vi "test-DiffDriveSim-convergence.vi"() -> (3 "Test Passed":bool)   [LabVIEW 2019]
uses:
  <vilib>/Rock Robotics/WPI/ThirdParty/JAS_Junk/TrajLib/DCMOTOR.CTL
  <vilib>/Rock Robotics/WPI/ThirdParty/JAS_Junk/TrajLib/LINEAR_SYSTEM.ctl
  <vilib>/Analysis/Matrix/Datatypes/RealMatrix.ctl
  <vilib>/Rock Robotics/WPI/ThirdParty/JAS_Junk/TrajLib/DIFF_DRIVE_TRAIN_SIM.ctl
  <vilib>/Rock Robotics/WPI/ThirdParty/JAS_Junk/TrajLib/POSE2D.ctl
  <vilib>/Rock Robotics/WPI/ThirdParty/JAS_Junk/TrajLib/TRANSLATION2D.ctl
  <vilib>/Rock Robotics/WPI/ThirdParty/JAS_Junk/TrajLib/ROTATION2D.ctl
  <vilib>/Rock Robotics/WPI/ThirdParty/JAS_Junk/TrajLib/DIFF_DRIVE_ToughBoxMini_MotorChoice_ENUM.ctl
  <vilib>/Rock Robotics/WPI/ThirdParty/JAS_Junk/TrajLib/TRAJECTORY_SPLINE_TYPE_ENUM.ctl
  <vilib>/Rock Robotics/WPI/ThirdParty/JAS_Junk/TrajLib/Translation2d_Create.vi
  <vilib>/Rock Robotics/WPI/ThirdParty/JAS_Junk/TrajLib/Rotation2d_CreateAngle.vi
  <vilib>/Rock Robotics/WPI/ThirdParty/JAS_Junk/TrajLib/MatBuilder_Create.vi
  <vilib>/Rock Robotics/SystemInterfaces/NetworkCommunication/NetComm_UsageReport_report.vi
  <vilib>/Rock Robotics/WPI/ThirdParty/JAS_Junk/TrajLib/DiffDriveKinematicsConstraint_New.vi
  <vilib>/Rock Robotics/WPI/ThirdParty/JAS_Junk/TrajLib/LinearSystem_New.vi
  <vilib>/Rock Robotics/WPI/ThirdParty/JAS_Junk/TrajLib/MatBuilder_Fill.vi
  <vilib>/Rock Robotics/WPI/ThirdParty/JAS_Junk/TrajLib/MatrixHelper_Zero.vi
  <vilib>/Rock Robotics/WPI/ThirdParty/JAS_Junk/TrajLib/Ramsete_New_B_Z.vi
  <vilib>/Rock Robotics/WPI/ThirdParty/JAS_Junk/TrajLib/Ramsete_SetTolerance.vi
  <vilib>/Rock Robotics/WPI/ThirdParty/JAS_Junk/TrajLib/Pose2d_New.vi
  <vilib>/Rock Robotics/WPI/ThirdParty/JAS_Junk/TrajLib/Conv_AngleRadians_Heading.vi
  <vilib>/Rock Robotics/WPI/ThirdParty/JAS_Junk/TrajLib/Ramsete_SetEnabled.vi
  <vilib>/Rock Robotics/WPI/ThirdParty/JAS_Junk/TrajLib/MatrixHelper_CoerceSize.vi
  <vilib>/Rock Robotics/WPI/ThirdParty/JAS_Junk/TrajLib/Util_LibraryGlobals.vi
  <vilib>/Rock Robotics/WPI/ThirdParty/JAS_Junk/TrajLib/DiffDriveTrainSim_GetDynamics.vi
  <vilib>/Rock Robotics/WPI/ThirdParty/JAS_Junk/TrajLib/Ramsete_Diff_DO_SI.vi
  <vilib>/Rock Robotics/WPI/ThirdParty/JAS_Junk/TrajLib/DiffWheel_Normalize.vi
  <vilib>/Rock Robotics/WPI/ThirdParty/JAS_Junk/TrajLib/Trajectory_Library.lvlib
  <vilib>/Analysis/Matrix/NI_Matrix.lvlib
panel:
  in  "Tab Control":T1(tab)
  out "SP Chart":T2(graph)
  out "XY Graph":cluster{dbl[], dbl[]}[](graph)
  out "Left Motor Vel (PV)":dbl format="%20.3f"
  out "Right Motor Vel (PV)":dbl format="%20.3f"
  out "Motor Amps":cluster{"Voltage":dbl}(graph)
  out "PV Chart":T2(graph)
  out "Motor Amps":dbl format="%20.3f"
  out "Sim Upd Err":bool
  out "Lin Sys Size Cooerced":bool
  out "AtReference":bool
  out "InvFF Error":bool
  out "SIM Pose":T3={"TRANSLATION"={"X"=0.0, "Y"=0.0}, "ROTATION"={"VALUE"=0.0, "COS"=1.0, "SIN"=0.0}} {"ROTATION"."SIN" format="%13.4f"; "ROTATION"."COS" format="%13.4f"; "ROTATION"."VALUE" format="%13.4f"; "TRANSLATION"."Y" format="%14.3f"; "TRANSLATION"."X" format="%14.3f"}
  out "m_Y":T6
  out "m_X":T6
  out "Ground Truth":T6
  out "RK4 Error":bool
  out "DiffDriveMotor":T7 {"Jr_KgM2" format="%13.5p"; "L_H" format="%13.5p"; "Kt_NMPerAmp" format="%13.5p"; "KvINV_RadPerSecPerVolt" format="%13.5p"; "R_Ohms" format="%13.5p"; "FreeSpeed_RadPerSec" format="%13.5p"; "FreeCurrent_Amps" format="%13.5p"; "StallCurrent_Amps" format="%13.5p"; "StallTorque_NM" format="%13.5p"; "nominalVoltage_Volts" format="%13.5p"}
  out "m_DiffDriveVel":T8
  out "Differential Drive Train Sim":T9 {"m_Motor"."Jr_KgM2" format="%13.5p"; "m_Motor"."L_H" format="%13.5p"; "m_Motor"."Kt_NMPerAmp" format="%13.5p"; "m_Motor"."KvINV_RadPerSecPerVolt" format="%13.5p"; "m_Motor"."R_Ohms" format="%13.5p"; "m_Motor"."FreeSpeed_RadPerSec" format="%13.5p"; "m_Motor"."FreeCurrent_Amps" format="%13.5p"; "m_Motor"."StallCurrent_Amps" format="%13.5p"; "m_Motor"."StallTorque_NM" format="%13.5p"; "m_Motor"."nominalVoltage_Volts" format="%13.5p"}
  # "<States,States>"
  # "<States,Inputs>"
  # "<Outputs,States>"
  # "<Outputs,Inputs>"
  # "<States, 1>"
  # "<Outputs, 1>"
  # "<Inputs, 1>"
  # "<Outputs, 1>"
  # "<States,States>"
  # "<States,Inputs>"
  # "<Outputs,States>"
  # "<Outputs,Inputs>"
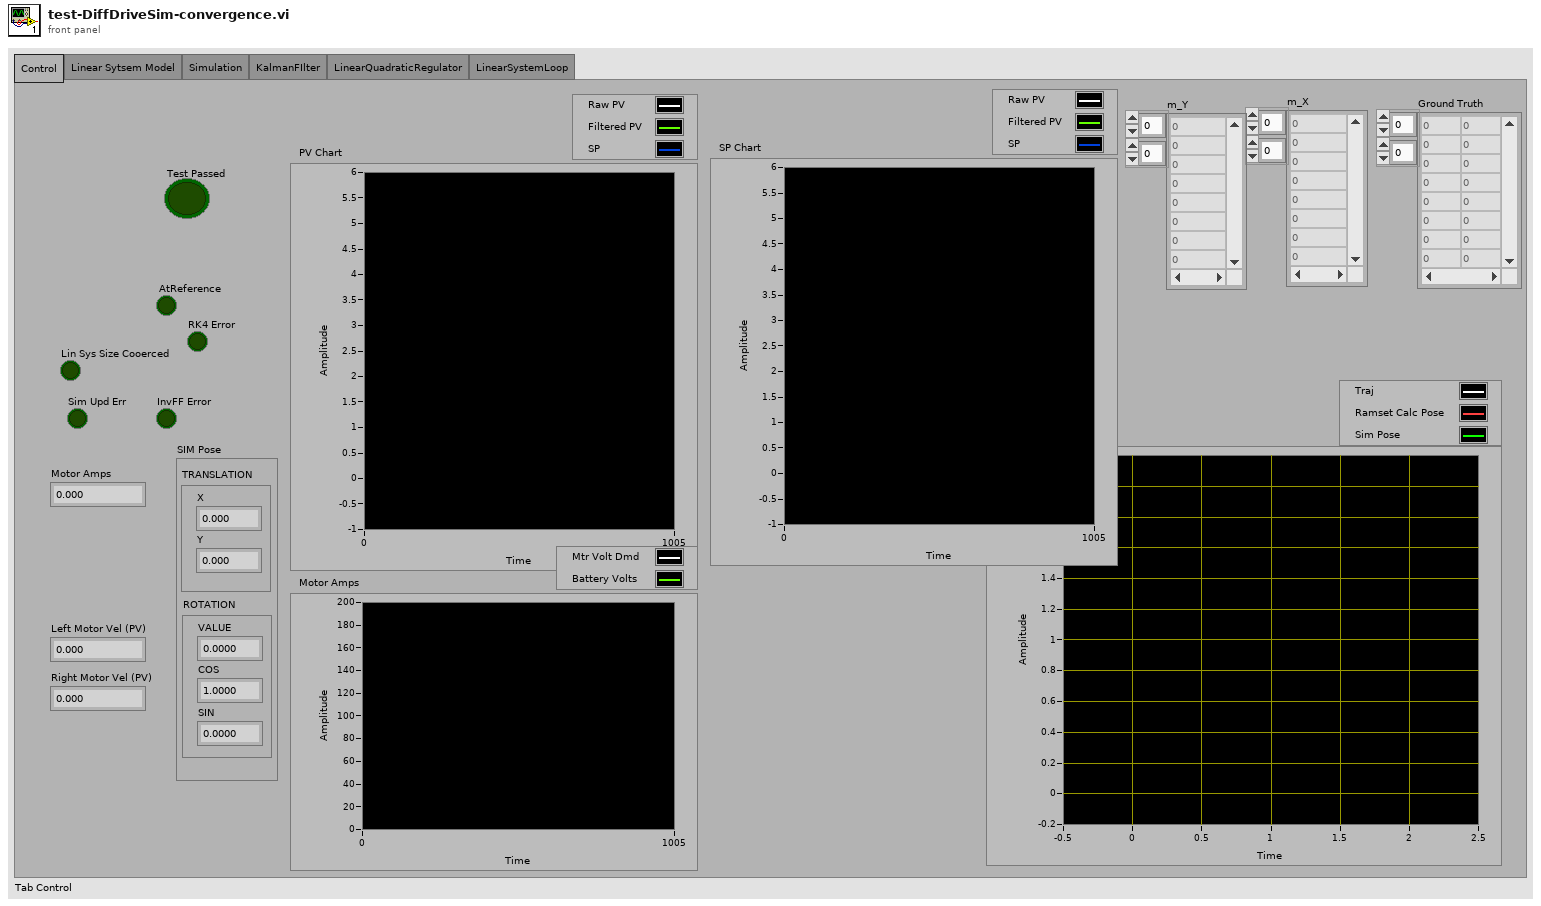
[diagram p1: front panel]
types:
  T1 = enum32{"Control", "Linear Sytsem Model", "Simulation", "KalmanFIlter", "LinearQuadraticRegulator", "LinearSystemLoop"}
  T2 = cluster{"LeftVelocity_M_Per_Sec":dbl, "RightVel_M_Per_Sec":dbl}
  T3 = typedef "Trajectory_Library.lvlib/POSE2D.ctl" = cluster{"TRANSLATION":T4, "ROTATION":T5}
  T4 = typedef "Trajectory_Library.lvlib/TRANSLATION2D.ctl" = cluster{"X":dbl, "Y":dbl}
  T5 = typedef "Trajectory_Library.lvlib/ROTATION2D.ctl" = cluster{"VALUE":dbl, "COS":dbl, "SIN":dbl}
  T6 = typedef "NI_Matrix.lvlib/RealMatrix.ctl" = dbl[][]
  T7 = typedef "Trajectory_Library.lvlib/DCMOTOR.CTL" = cluster{"nominalVoltage_Volts":dbl, "StallTorque_NM":dbl, "StallCurrent_Amps":dbl, "FreeCurrent_Amps":dbl, "FreeSpeed_RadPerSec":dbl, "R_Ohms":dbl, "KvINV_RadPerSecPerVolt":dbl, "Kt_NMPerAmp":dbl, "L_H":dbl, "Jr_KgM2":dbl}
  T8 = typedef "Trajectory_Library.lvlib/LINEAR_SYSTEM.ctl" = cluster{"m_A":T6, "m_B":T6, "m_C":T6, "m_D":T6, "States":i32, "Inputs":i32, "Outputs":i32}
  T9 = typedef "Trajectory_Library.lvlib/DIFF_DRIVE_TRAIN_SIM.ctl" = cluster{"m_Plant":T8, "m_X":T6, "m_Y":T6, "m_U":T6, "MeasureStdDev":T6, "m_Motor":T7, "m_OriginalGearing":dbl, "m_CurrentGearing":dbl, "m_WheelRadius_M":dbl, "m_RB":dbl}
  T10 = typedef "Trajectory_Library.lvlib/TRAJECTORY_SPLINE_TYPE_ENUM.ctl" = enum16{"Cubic", "Cubic With Weights", "Quintic", "Quintic With Weights"}
  T11 = typedef "Trajectory_Library.lvlib/DIFF_DRIVE_ToughBoxMini_MotorChoice_ENUM.ctl" = enum16{"One CIM Per Side", "Two CIM Per Side", "One MiniCIM Per Side", "Two Mini CIM Per Side", "Two Falcon Per Side", "Two NEO Per Side"}
  T12 = typedef "Trajectory_Library.lvlib/TRAJ_CONFIG.ctl" = cluster{"MaxVelocity":dbl, "Max Acceleration":dbl, "StartVelocity":dbl, "End Velocity":dbl, "Reversed":bool, "DiffDrKineConstntDefined":bool, "CentAcellConstntDefined":bool, "DiffDrVoltConstntDefined":bool, "DIFF_DRIVE_KINE_CONSTRAINT":T13, "CENTRIPETAL_ACCEL_CONSTRAINT":T15, "SwerveDrKineConstntDefined":bool, "SWERVE_DRIVE_KINE_CONSTRAINT":T16, "DIFF_DRIVE_VOLTAGE_CONSTRAINT":T18, "MECANUM_DRIVE_KINE_CONSTRAINT":T20, "MecanumDrKineConstntDefined":bool}
  T13 = typedef "Trajectory_Library.lvlib/TRAJ_CONSTRAINT_DIIF_DRIVE_KINEMATICS.ctl" = cluster{"Max Speed (M/S)":dbl, "DIFF_DRIVE_KINEMATICS":T14, "Max Accel (M/S2)":dbl}
  T14 = typedef "Trajectory_Library.lvlib/DIFF_DRIVE_KINEMATICS.ctl" = cluster{"TrackWidth_Meters":dbl}
  T15 = typedef "Trajectory_Library.lvlib/TRAJ_CONSTRAINT_CENTRIPETAL_ACCEL.ctl" = cluster{"Max Cent Accel":dbl}
  T16 = typedef "Trajectory_Library.lvlib/TRAJ_CONSTRAINT_SWERVE_DRIVE_KINEMATICS.ctl" = cluster{"Max Speed (M/S)":dbl, "SwerveKinematics":T17}
  T17 = typedef "Trajectory_Library.lvlib/SWERVE_DRIVE_KINEMATICS.ctl" = cluster{"NumModules":i32, "InverseKinematics":T6, "ForwardKinematics":T6, "Modules":T4[], "PrevCoR":T4}
  T18 = typedef "Trajectory_Library.lvlib/TRAJ_CONSTRAINT_DIIF_DRIVE_VOLTAGE.ctl" = cluster{"Max Voltage":dbl, "DIFF_DRIVE_KINEMATICS":T14, "SIMPLE_MOTOR_FF":T19}
  T19 = typedef "Trajectory_Library.lvlib/SIMPLE_MOTOR_FF.ctl" = cluster{"Ks":dbl, "Kv":dbl, "Ka":dbl}
  T20 = typedef "Trajectory_Library.lvlib/TRAJ_CONSTRAINT_MECA_DRIVE_KINEMATICS.ctl" = cluster{"Max Speed (M/S)":dbl, "MECA_DRIVE_KINEMATICS":T21}
  T21 = typedef "Trajectory_Library.lvlib/MECA_DRIVE_KINEMATICS.ctl" = cluster{"FrontLeft":T4, "FrontRight":T4, "RearLeft":T4, "RearRight":T4, "InverseKinematics":T6, "ForwardKinematics":T6, "PrevCoR":T4}
  T22 = typedef "Trajectory_Library.lvlib/WEIGHTED_WAYPOINT.ctl" = cluster{"TRANSLATION":T4, "ROTATION":T5, "SCALAR":dbl}
  T23 = typedef "Trajectory_Library.lvlib/TRAJECTORY.ctl" = cluster{"TotalTImeSecs":dbl, "States":T24[]}
  T24 = typedef "Trajectory_Library.lvlib/TRAJ_STATE.ctl" = cluster{"TimeSeconds":dbl, "Velocity":dbl, "Acceleration":dbl, "POSE":T3, "Curvature":dbl}
  T25 = typedef "Trajectory_Library.lvlib/LINEAR_PLANT_INV_FF.ctl" = cluster{"m_R":T6, "m_Uff":T6, "m_B":T6, "m_A":T6, "States":i32, "Inputs":i32}
  T26 = typedef "Trajectory_Library.lvlib/RAMSETE_EXE_TUNING.ctl" = cluster{"B":dbl, "Zeta":dbl, "X Tolerance M":dbl, "Y Tolerance M":dbl, "Heading Tolerance RAD":dbl, "Track Width M":dbl, "Max Speed M/S":dbl}
  T27 = cluster{"Left Speed Dmd M/S":dbl, "Right Speed Dmd M/S":dbl}
  T28 = cluster{"m_A":T6, "m_B":T6, "m_CurrentGearing":dbl, "m_OriginalGearing":dbl, "m_RB":dbl}
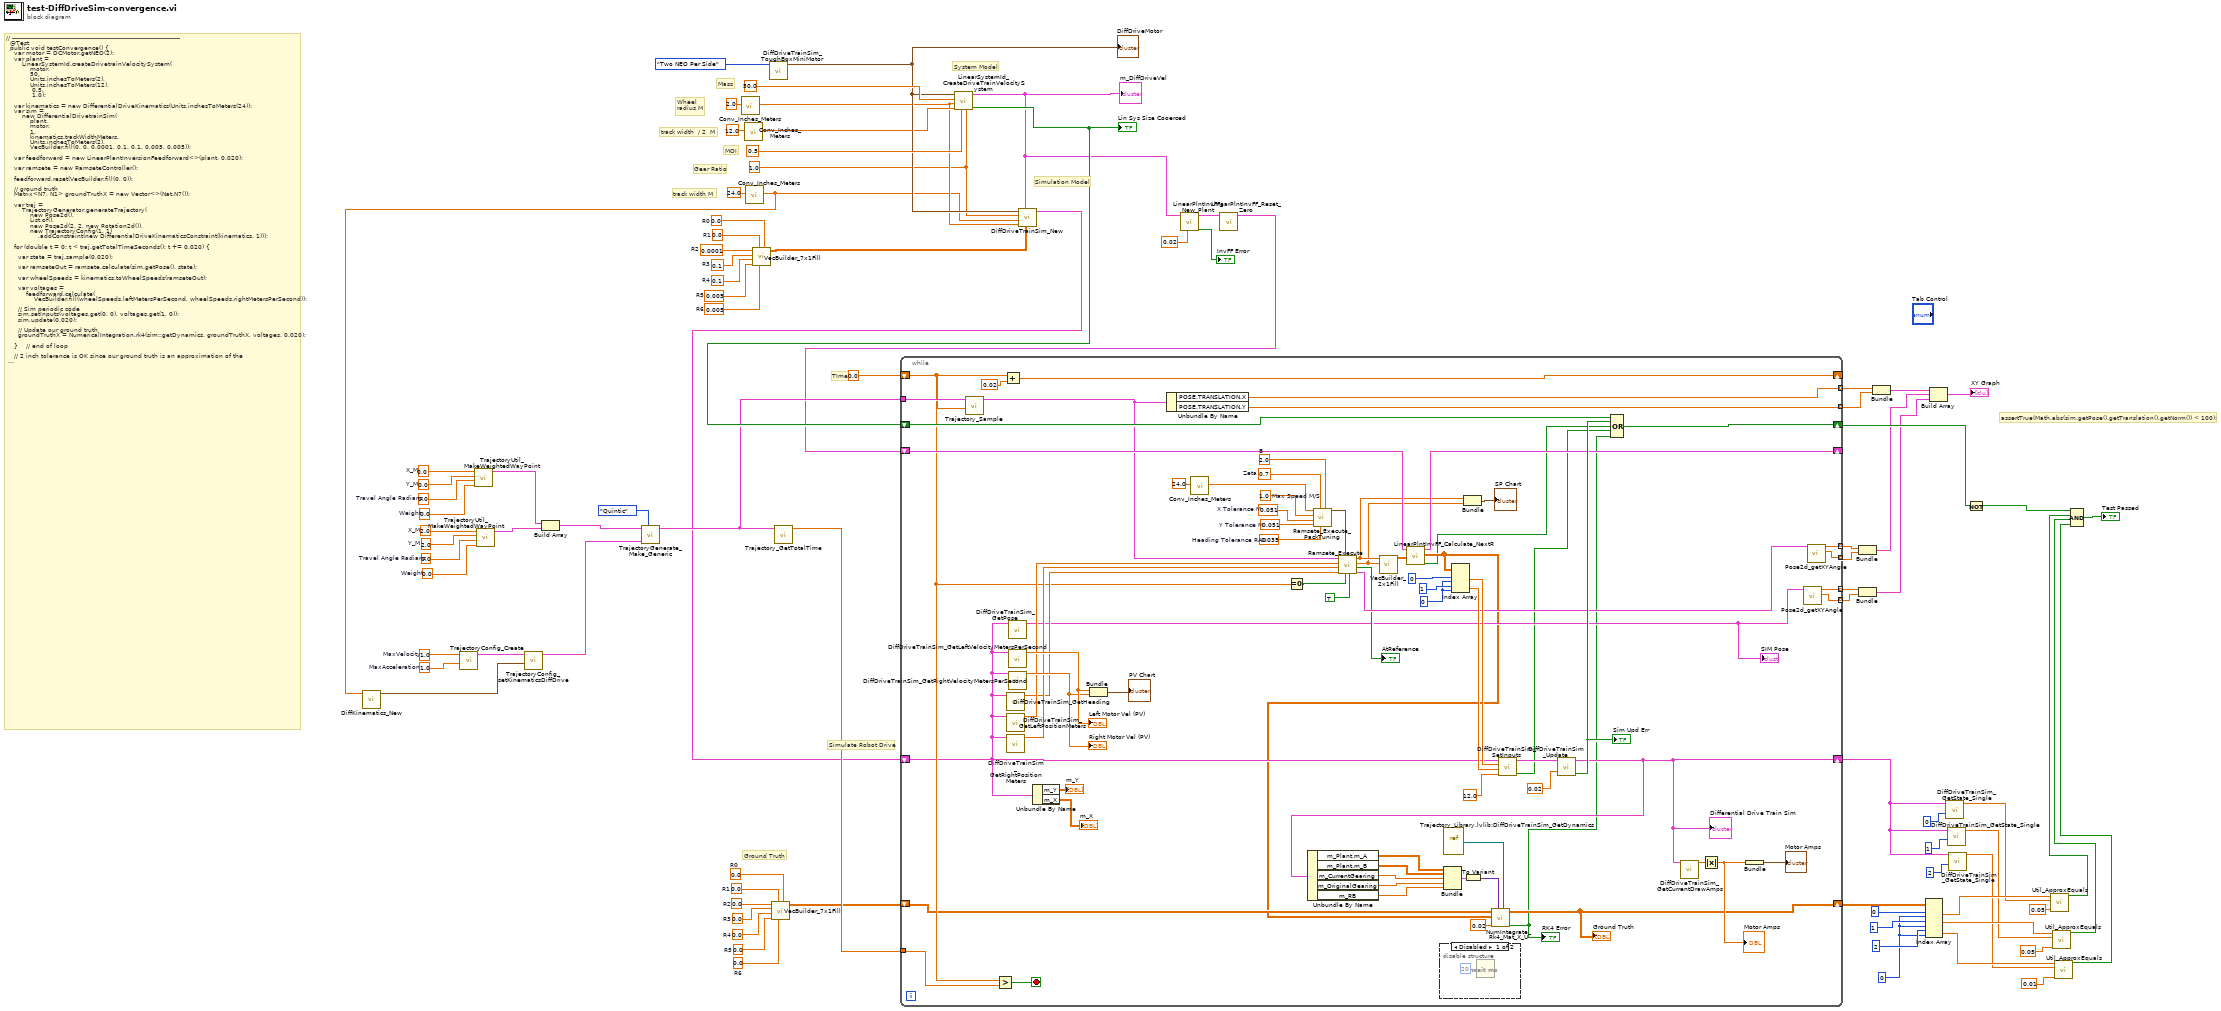
[diagram p0: block diagram]
diagram:
  w17 = 0 ("index (col)")
  w58 = 2.0  # X_M
  w57 = 2.0  # Y_M
  w56 = 0.0  # Travel Angle Radians
  w55 = 0.0  # Weight
  w54 = 0.0  # X_M
  w53 = 0.0  # Y_M
  w52 = 0.0  # Travel Angle Radians
  w51 = 0.0  # Weight
  w50 = 1.0  # MaxVelocity
  w49 = 1.0  # MaxAcceleration
  w66 = 0.0  # R6
  w65 = 0.0  # R5
  w64 = 0.0  # R4
  w63 = 0.0  # R3
  w62 = 0.0  # R2
  w61 = 0.0  # R1
  w60 = 0.0  # R0
  w78 = 0.005  # R6
  w77 = 0.005  # R5
  w76 = 0.1  # R4
  w75 = 0.1  # R3
  w74 = 0.0001  # R2
  w73 = 0.0  # R1
  w72 = 0.0  # R0
  w80 = 1.0 ("G")
  # "TIme"
  # "Ground Truth"
  # "// ------------------------------------------------------------------------------------\n  @Test\n  public void testConvergence() {\n    var motor = DCMotor.getNEO(2);\n    var plant =\n        LinearSystemId.createDrivetrainVelocitySystem(\n            motor, \n            50, \n            Units.inchesToMeters(2), \n            Units.inchesToMeters(12), \n             0.5, \n             1.0);\n\n    var kinematics = new DifferentialDriveKinematics(Units.inchesToMeters(24));\n    var sim =\n        new DifferentialDrivetrainSim(\n            plant,\n            motor,\n            1,\n            kinematics.trackWidthMeters,\n            Units.inchesToMeters(2),\n            VecBuilder.fill(0, 0, 0.0001, 0.1, 0.1, 0.005, 0.005));\n\n    var feedforward = new LinearPlantInversionFeedforward<>(plant, 0.020);\n\n    var ramsete = new RamseteController();\n\n    feedforward.reset(VecBuilder.fill(0, 0));\n\n    // ground truth\n    Matrix<N7, N1> groundTruthX = new Vector<>(Nat.N7());\n\n    var traj =\n        TrajectoryGenerator.generateTrajectory(\n            new Pose2d(),\n            List.of(),\n            new Pose2d(2, 2, new Rotation2d()),\n            new TrajectoryConfig(1, 1)\n                .addConstraint(new DifferentialDriveKinematicsConstraint(kinematics, 1)));\n\n    for (double t = 0; t < traj.getTotalTimeSeconds(); t += 0.020) {\n\n      var state = traj.sample(0.020);\n\n      var ramseteOut = ramsete.calculate(sim.getPose(), state);\n\n      var wheelSpeeds = kinematics.toWheelSpeeds(ramseteOut);\n\n      var voltages =\n          feedforward.calculate(\n              VecBuilder.fill(wheelSpeeds.leftMetersPerSecond, wheelSpeeds.rightMetersPerSecond));\n\n      // Sim periodic code\n      sim.setInputs(voltages.get(0, 0), voltages.get(1, 0));\n      sim.update(0.020);\n\n      // Update our ground truth\n      groundTruthX = NumericalIntegration.rk4(sim::getDynamics, groundTruthX, voltages, 0.020);\n\n    }    // end of loop\n\n    // 2 inch tolerance is OK since our ground truth is an approximation of the\n    // ODE solution using RK4 anyway\n    assertEquals(\n        groundTruthX.get(DifferentialDrivetrainSim.State.kX.value, 0),\n        sim.getState(DifferentialDrivetrainSim.State.kX),\n        0.05);\n    assertEquals(\n        groundTruthX.get(DifferentialDrivetrainSim.State.kY.value, 0),\n        sim.getState(DifferentialDrivetrainSim.State.kY),\n        0.05);\n    assertEquals(\n        groundTruthX.get(DifferentialDrivetrainSim.State.kHeading.value, 0),\n        sim.getState(DifferentialDrivetrainSim.State.kHeading),\n        0.01);\n  }\n\n\n}"
  # "assertTrue(Math.abs(sim.getPose().getTranslation().getNorm()) < 100);"
  # "track width M"
  # "Gear Ratio"
  # "Wheel\nradius M"
  # "track width  / 2  M"
  # "MOI"
  # "Simulation Model"
  # "System Model"
  # "Mass"
  # "Simulate Robot Drive"
  n1 = call <vilib>:"TrajectoryConfig_Create.vi"("MaxAcceleration"=w49, "MaxVelocity"=w50) -> ("TRAJECTORY_CONFIG"=w43:T12)  [unwired: 9 in]
  n2 = call <vilib>:"TrajectoryUtil_MakeWeightedWayPoint.vi"("Weight"=w51, "Travel Angle Radians"=w52, "Y_M"=w53, "X_M"=w54) -> ("WEIGHTED_WAYPOINT"=w46:T22)  [unwired: 7 in]
  n3 = call <vilib>:"TrajectoryUtil_MakeWeightedWayPoint.vi"("Weight"=w55, "Travel Angle Radians"=w56, "Y_M"=w57, "X_M"=w58) -> ("WEIGHTED_WAYPOINT"=w59:T22)  [unwired: 7 in]
  n4 = Build Array(w46, w59) -> (w47:T22[])
  n5 = call <vilib>:"Conv_Inches_Meters.vi"("INCH"=2.0) -> ("Meters"=w81:dbl)  [unwired: 10 in]
  n6 = call <vilib>:"Conv_Inches_Meters.vi"("INCH"=12.0) -> ("Meters"=w82:dbl)  [unwired: 10 in]
  n7 = call <vilib>:"Conv_Inches_Meters.vi"("INCH"=24.0) -> ("Meters"=w45:dbl)  [unwired: 10 in]
  n8 = call <vilib>:"DiffKinematics_New.vi"("TrackWidth_Meters"=w45) -> ("DIFF_DRIVE_KINEMATICS"=w44:T14)  [unwired: 10 in]
  n9 = call <vilib>:"TrajectoryConfig_setKinematicsDiffDrive.vi"("DIFF_DRIVE_KINEMATICS"=w44, "inTRAJECTORY_CONFIG"=w43) -> ("outTRAJECTORY_CONFIG"=w42:T12)  [unwired: 9 in]
  n10 = call <vilib>:"TrajectoryGenerate_Make_Generic.vi"("Spline Type"=TRAJECTORY_SPLINE_TYPE_ENUM."Quintic", "traj_config"=w42, "WeightedWayPoints"=w47) -> ("TRAJECTORY"=w36:T23)  [unwired: 7 in, 1 out]
  n11 = call <vilib>:"VecBuilder_7x1Fill.vi"("R0"=w72, "R6"=w78, "R1"=w73, "R5"=w77, "R4"=w76, "R3"=w75, "R2"=w74) -> ("output matrix"=w71:T6)  [unwired: 4 in]
  n12 = call <vilib>:"DiffDriveTrainSim_ToughBoxMiniMotor.vi"("ToughBoxMiniMotor"=DIFF_DRIVE_ToughBoxMini_MotorChoice_ENUM."Two NEO Per Side") -> ("DriveMotor"=w83:T7)  [unwired: 10 in]
  "DiffDriveMotor" <- w83
  n13 = call <vilib>:"VecBuilder_7x1Fill.vi"("R0"=w60, "R6"=w66, "R1"=w61, "R5"=w65, "R4"=w64, "R3"=w63, "R2"=w62) -> ("output matrix"=w22:T6)  [unwired: 4 in]
  n14 = call <vilib>:"Trajectory_GetTotalTime.vi"("TRAJECTORY"=w36) -> ("TotalTime_Sec"=w35:dbl)  [unwired: 10 in]
  n15 = call <vilib>:"LinearSystemId_CreateDriveTrainVelocitySystem.vi"("G"=w80, "JKgMetersSquared"=0.5 ("Mass_Kg"), "rbMeters"=w82, "rMeters"=w81, "MassKg"=50.0 ("Mass_Kg"), "Motor"=w83) -> ("Size Coerced"=w70:bool, "Linearsystem"=w40:T8)  [unwired: 4 in]
  "m_DiffDriveVel" <- w40
  "Lin Sys Size Cooerced" <- w70
  n16 = call <vilib>:"DiffDriveTrainSim_New.vi"("MeasurementStdDev"=w71, "DriveTrainPlant"=w40, "WheelRadius_M"=w81, "TrackWidth_M"=w45, "Gearing"=w80, "DriveMotor"=w83) -> ("DiffDriveTrainSim"=w33:T9)  [unwired: 5 in]
  n17 = call <vilib>:"LinearPlntInvFF_New_Plant.vi"("dT_Seconds"=0.02, "Plant"=w40) -> ("Error"=→"InvFF Error":bool, "Linear Plnt Inversion FF"=w38:T25)  [unwired: 8 in]
  n18 = call <vilib>:"LinearPlntInvFF_Reset_Zero.vi"("Input Linear Plant Inv FF"=w38) -> ("Output Linear Plant Inv FF"=w34:T25)  [unwired: 10 in]
  n19 = while {
    shift-right: [w104] -> w7
    shift-left: w33 -> [w107]
    shift-right: [w150] -> w69
    shift-left: w70 -> [w151]
    tunnel: w36 -> [w139]
    shift-right: [w147] -> _
    shift-left: 0.0 -> [w115]
    tunnel: w35 -> [w149]
    shift-right: [w133] -> _
    shift-left: w34 -> [w135]
    tunnel: [w124] -> w32 mode=indexing
    tunnel: [w123] -> w31 mode=indexing
    tunnel: [w122] -> w30 mode=indexing
    tunnel: [w121] -> w29 mode=indexing
    tunnel: [w109] -> w25 mode=indexing
    tunnel: [w108] -> w24 mode=indexing
    shift-right: [w92] -> w21
    shift-left: w22 -> [w95]
    stop <- w156 stop-if-true
    w128 = 0 ("index (col)")
    w146 = 1.0  # Max Speed M/S
    w145 = 0.051  # X Tolerance M
    w144 = 0.051  # Y Tolerance M
    w143 = 0.7  # Zeta
    w142 = 0.035  # Heading Tolerance RAD
    w141 = 2.0  # B
    n20 = call <vilib>:"Trajectory_Sample.vi"("Time"=w115, "InputTRAJECTORY"=w139) -> ("OutputTRAJ_STATE"=w125:T24)  [unwired: 9 in]
    n21 = Greater?(x=w115, y=w149) -> (0:w156:bool)
    n22 = Add(x=w115, y=0.02) -> (x+y=w147:dbl)
    n23 = call <vilib>:"DiffDriveTrainSim_GetHeading.vi"("DiffDriveTrainSim"=w107) -> ("Heading"=w136:dbl)  [unwired: 10 in]
    n24 = call <vilib>:"DiffDriveTrainSim_GetLeftPositionMeters.vi"("DiffDriveTrainSim"=w107) -> ("LeftPosition_Meters"=w138:dbl)  [unwired: 10 in]
    n25 = call <vilib>:"DiffDriveTrainSim_GetRightPositionMeters.vi"("DiffDriveTrainSim"=w107) -> ("RightPosition_Meters"=w137:dbl)  [unwired: 10 in]
    n26 = call <vilib>:"DiffDriveTrainSim_GetRightVelocityMetersPerSecond.vi"("DiffDriveTrainSim"=w107) -> ("RightVel_M_Per_Sec"=w154:dbl)  [unwired: 10 in]
    "Right Motor Vel (PV)" <- w154
    n27 = call <vilib>:"DiffDriveTrainSim_GetPose.vi"("DiffDriveTrainSim"=w107) -> ("Pose"=w110:T3)  [unwired: 10 in]
    "SIM Pose" <- w110
    n28 = call <vilib>:"DiffDriveTrainSim_GetLeftVelocityMetersPerSecond.vi"("DiffDriveTrainSim"=w107) -> ("LeftVelocity_M_Per_Sec"=w158:dbl)  [unwired: 10 in]
    "Left Motor Vel (PV)" <- w158
    n29 = Unbundle By Name(w107) -> ("m_Y"=→"m_Y":T6, "m_X"=→"m_X":T6)
    n30 = Bundle("LeftVelocity_M_Per_Sec"=w158, "RightVel_M_Per_Sec"=w154) -> (→"PV Chart":T2)  [unwired: 1 in]
    n31 = Unbundle By Name(w125) -> ("POSE.TRANSLATION.X"=w124:dbl, "POSE.TRANSLATION.Y"=w123:dbl)
    n32 = call <vilib>:"Conv_Inches_Meters.vi"("INCH"=24.0) -> ("Meters"=w113:dbl)  [unwired: 10 in]
    n33 = Equal To 0?(x=w115) -> (x = 0?=w116:bool)
    n34 = call <vilib>:"Ramsete_Execute_PackTuning.vi"("B"=w141, "Heading Tolerance RAD"=w142, "Zeta"=w143, "Y Tolerance M"=w144, "X Tolerance M"=w145, "Max Speed M/S"=w146, "Track Width M"=w113) -> ("RAMSETE_EXE_TUNING"=w140:T26)  [unwired: 4 in]
    n35 = call <vilib>:"Ramsete_Execute.vi"("Enabled"=TRUE, "Reset"=w116, "RAMSETE_EXE_TUNING"=w140, "Gyro-Radians\n(Inc counterclockwise)"=w136, "RightDist-Meters"=w137, "LeftDist-Meters"=w138, "TRAJ_STATE"=w125) -> ("CurrentRelativePose"=w112:T3, "AtReference"=→"AtReference":bool, "Right Speed Dmd M/S"=w118:dbl, "Left Speed Dmd M/S"=w119:dbl)  [unwired: 1 out]
    n36 = call <vilib>:"VecBuilder_2x1Fill.vi"("R1"=w118, "R0"=w119) -> ("output matrix"=w134:T6)  [unwired: 9 in]
    n37 = call <vilib>:"LinearPlntInvFF_Calculate_NextR.vi"("NextR"=w134, "Input Linear Plant Inv FF"=w135) -> ("Error"=w91:bool, "Uff"=w94:T6, "Output Linear Plant Inv FF"=w133:T25)  [unwired: 7 in]
    n38 = disable-structure shown="Disabled" {
      frame Disabled {
        n39 = Wait (ms)(milliseconds to wait=u32 20) -> ()  [unwired: 1 out]
      }
      frame Enabled {
      }
    }
    n40 = vi-ref "Trajectory_Library.lvlib:DiffDriveTrainSim_GetDynamics.vi"() -> (w96:refnum<vi>)
    n41 = Index Array(array=w94, index (row) #1=0 ("index (row)"), index (col) #1=w128, index (row) #2=1 ("index (row)"), index (col) #2=w128) -> (element #1=w127:dbl, element #2=w126:dbl)
    n42 = Bundle("Left Speed Dmd M/S"=w119, "Right Speed Dmd M/S"=w118) -> (→"SP Chart":T27)  [unwired: 1 in]
    n43 = call <vilib>:"DiffDriveTrainSim_SetInputs.vi"("BatteryVoltage"=12.0, "Right_Volts"=w126, "Left_Volts"=w127, "in DiffDriveTrainSim"=w107) -> ("Size Coerced"=w90:bool, "out DiffDriveTrainSim"=w131:T9)  [unwired: 6 in]
    n44 = call <vilib>:"DiffDriveTrainSim_Update.vi"("dT_Seconds"=0.02, "in DiffDriveTrainSim"=w131) -> ("Error"=w152:bool, "out DiffDriveTrainSim"=w104:T9)  [unwired: 8 in]
    "Sim Upd Err" <- w152
    "Differential Drive Train Sim" <- w104
    n45 = Unbundle By Name(w104) -> ("m_Plant.m_A"=w103:T6, "m_Plant.m_B"=w102:T6, "m_CurrentGearing"=w101:dbl, "m_OriginalGearing"=w100:dbl, "m_RB"=w99:dbl)
    n46 = Bundle("m_A"=w103, "m_B"=w102, "m_CurrentGearing"=w101, "m_OriginalGearing"=w100, "m_RB"=w99) -> (w98:T28)  [unwired: 1 in]
    n47 = To Variant(anything=w98) -> (Variant=w97:variant)
    n48 = call <vilib>:"NumIntegrate_Rk4_Mat_X_U.vi"("Func_X_U_Extra"=w96, "PassedData"=w97, "dT_Seconds"=0.02, "U"=w94, "X"=w95) -> ("Error"=w89:bool, "OUTPUT"=w92:T6)  [unwired: 5 in]
    "RK4 Error" <- w89
    "Ground Truth" <- w92
    n49 = Compound Arithmetic op=OR(w151, w152, w91, w90, w89) -> (w150:bool)
    n50 = call <vilib>:"DiffDriveTrainSim_GetCurrentDrawAmps.vi"("DiffDriveTrainSim"=w104) -> ("TotalCurrent_Amps"=w159:dbl)  [unwired: 10 in]
    n51 = Absolute Value(x=w159) -> (abs(x)=w155:dbl)
    "Motor Amps" <- w155
    n52 = Bundle(w155) -> (→"Motor Amps":cluster{dbl})  [unwired: 1 in]
    n53 = call <vilib>:"Pose2d_getXYAngle.vi"("in POSE"=w110) -> ("Y"=w108:dbl, "X"=w109:dbl)  [unwired: 8 in, 1 out]
    n54 = call <vilib>:"Pose2d_getXYAngle.vi"("in POSE"=w112) -> ("Y"=w121:dbl, "X"=w122:dbl)  [unwired: 8 in, 1 out]
  }
  n55 = Bundle(w30, w29) -> (w27:cluster{dbl[], dbl[]})  [unwired: 1 in]
  n56 = Bundle(w25, w24) -> (w23:cluster{dbl[], dbl[]})  [unwired: 1 in]
  n57 = Bundle(w32, w31) -> (w28:cluster{dbl[], dbl[]})  [unwired: 1 in]
  n58 = Index Array(array=w21, index (row) #1=0 ("index (row)"), index (col) #1=w17, index (row) #2=1 ("index (row)"), index (col) #2=w17, index (row) #3=2 ("index (row)"), index (col) #3=w17) -> (element #1=w16:dbl, element #2=w12:dbl, element #3=w11:dbl)
  n59 = Build Array(w28, w27, w23) -> (→"XY Graph":cluster{dbl[], dbl[]}[])
  n60 = call <vilib>:"DiffDriveTrainSim_GetState_Single.vi"("Row"=0, "DiffDriveTrainSim"=w7) -> ("State"=w6:dbl)  [unwired: 9 in]
  n61 = call <vilib>:"DiffDriveTrainSim_GetState_Single.vi"("Row"=1, "DiffDriveTrainSim"=w7) -> ("State"=w5:dbl)  [unwired: 9 in]
  n62 = call <vilib>:"DiffDriveTrainSim_GetState_Single.vi"("Row"=2, "DiffDriveTrainSim"=w7) -> ("State"=w4:dbl)  [unwired: 9 in]
  n63 = Not(x=w69) -> (.not. x?=w68:bool)
  n64 = call <vilib>:"Util_ApproxEquals.vi"("Tolerance"=0.05, "Value 2"=w6, "Value 1"=w16) -> ("ApproxEquals"=w3:bool)  [unwired: 8 in]
  n65 = call <vilib>:"Util_ApproxEquals.vi"("Tolerance"=0.05, "Value 2"=w5, "Value 1"=w12) -> ("ApproxEquals"=w2:bool)  [unwired: 8 in]
  n66 = call <vilib>:"Util_ApproxEquals.vi"("Tolerance"=0.01, "Value 2"=w4, "Value 1"=w11) -> ("ApproxEquals"=w1:bool)  [unwired: 8 in]
  n67 = Compound Arithmetic op=AND(w68, w3, w2, w1) -> (→"Test Passed":bool)
